vi "menuActivate.vi"(8 "error in (no error)":errorcluster, 10 "flatMenu[] in":T1, 11 "Packet in":refnum<class "Packet.lvclass">) -> (0 "error out":errorcluster, 2 "flatMenu[] out":T1, 3 "Packet out":refnum<class "Packet.lvclass">)   [LabVIEW 2013, in "Packet.lvclass"]
doc: "Takes the relevent data of the xceDataNode, and produces an array which represents the menu options in the tree control."
uses:
  Packet.lvclass
  xCE/_shared/flatMenu.ctl
  xCE/xceDataNode/xceDataNode.lvclass
  Packet.lvclass/Packet.ctl
  Channel/Channel.lvclass
  xCE/xceNode/xceNode.lvclass
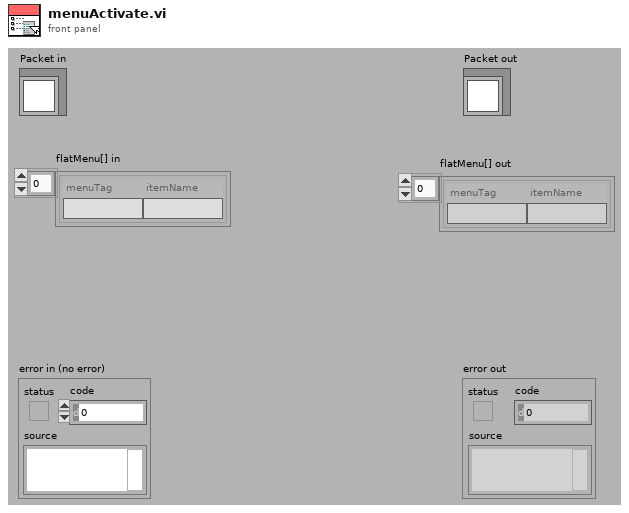
[diagram p1: front panel]
types:
  T1 = typedef "flatMenu.ctl" = cluster{"menuTag":string, "itemName":string}[]
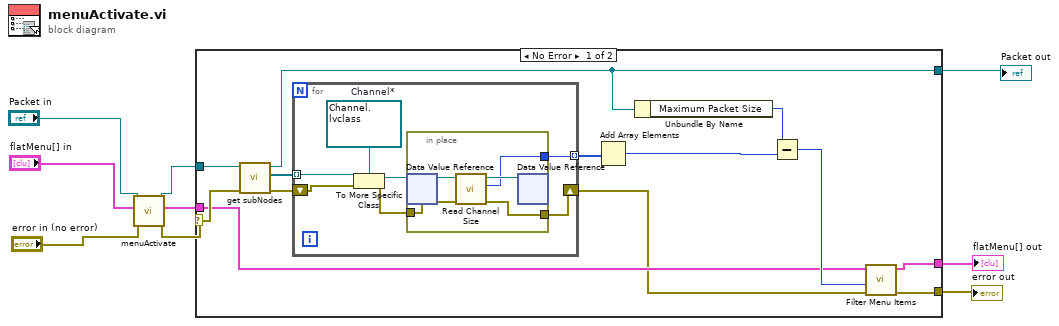
[diagram p0: block diagram]
diagram:
  n1 = call-parent "menuActivate.vi"("error in (no error)"="error in (no error)", "flatMenu[] in"="flatMenu[] in", "xceDataNode in"="Packet in") -> ("error out"=w6:errorcluster, "flatMenu[] out"=w5:T1, "xceDataNode out"=w4:refnum<class "Packet.lvclass">)  [unwired: 6 in]
  n2 = case shown="No Error" w6 {
    selector: w6 -> [w21 w35]
    tunnel: w5 -> [w13 w36]
    tunnel: w4 -> [w22 w37]
    tunnel: [w15 w37] -> w1
    tunnel: [w10 w36] -> w2
    tunnel: [w11 w35] -> w3
    frame No Error {
      n3 = call "get subNodes.vi"("error in (no error)"=w21, "xceNode in"=w22) -> ("error out"=w19:errorcluster, "subNodes[]*"=w20:refnum<data-value>[], "xceNode out"=w15:refnum<class "Packet.lvclass">)  [unwired: 7 in]
      n4 = for {
        tunnel: w20 -> [w28] mode=indexing
        shift-right: [w24] -> w12
        shift-left: w19 -> [w27]
        tunnel: [w23] -> w18 mode=indexing
        w29 = refnum<data-value> refnum  # Channel*
        n5 = To More Specific Class(target class=w29, reference=w28, error in=w27) -> (specific class reference=w26:refnum<data-value>, error out=w25:errorcluster)
        n6 = in-place {
          in-place-border: w25 -> [w33]
          in-place-border: [w32] -> w24
          in-place-border: [w30] -> w23
          n7 = in-place-dvr #1(w26) -> (w34:refnum<class "Channel.lvclass">)  [unwired: 1 out]
          n8 = call "Read Channel Size.vi"("error in (no error)"=w33, "Channel in"=w34) -> ("error out"=w32:errorcluster, "Channel Size"=w30:i32, "Channel out"=w31:refnum<class "Channel.lvclass">)  [unwired: 7 in]
          n9 = in-place-dvr #1(w31) -> ()  [unwired: 2 out]
        }
      }
      n10 = Add Array Elements(numeric array=w18) -> (sum=w16:i32)
      n11 = Unbundle By Name(w15) -> ("Maximum Packet Size"=w17:i32)
      n12 = Subtract(x=w17, y=w16) -> (x-y=w14:i32)
      n13 = call "Filter Menu Items.vi"("error in (no error)"=w12, "Bit threshold"=w14, "flatMenu[] in"=w13) -> ("error out"=w11:errorcluster, "flatMenu[] out"=w10:T1)  [unwired: 7 in]
    }
    frame Error {
    }
  }
  "error out" <- w3
  "flatMenu[] out" <- w2
  "Packet out" <- w1
